vi "Write Parameters.vi"(8 "error in (no error)":errorcluster, 10 "Parameters":T1, 11 "PID in":refnum<class "PID.lvclass">) -> (0 "error out":errorcluster, 3 "PID out":refnum<class "PID.lvclass">)   [LabVIEW 2020, in "IG PID.lvlib" / "PID.lvclass"]
uses:
  PID.lvclass
  Parameters.ctl
  PID.lvclass/PID.ctl
  IG PID.lvlib
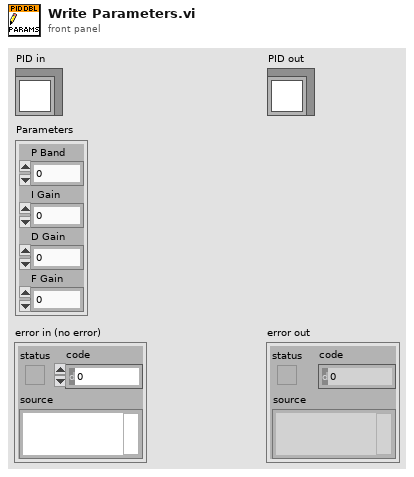
[diagram p1: front panel]
types:
  T1 = typedef "IG PID.lvlib/Parameters.ctl" = cluster{"P Band":dbl, "I Gain":dbl, "D Gain":dbl, "F Gain":dbl}
  T2 = typedef "IG PID.lvlib/Output Range.ctl" = cluster{"Min":dbl, "Max":dbl}
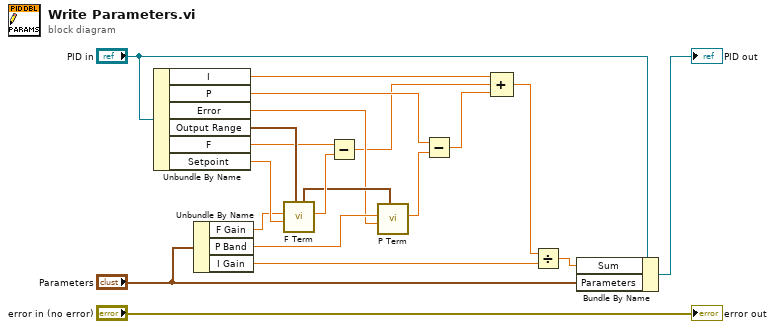
[diagram p0: block diagram]
diagram:
  n1 = Unbundle By Name("PID in") -> ("I"=w15:dbl, "P"=w3:dbl, "Error"=w5:dbl, "Output Range"=w10:T2, "F"=w9:dbl, "Setpoint"=w12:dbl)
  n2 = Unbundle By Name("Parameters") -> ("F Gain"=w11:dbl, "P Band"=w6:dbl, "I Gain"=w13:dbl)
  n3 = call "F Term.vi"("Output Range"=w10, "Setpoint"=w12, "F Gain"=w11) -> ("Output"=w8:dbl, "Remaining Range"=w7:T2)  [unwired: 7 in]
  n4 = Subtract(x=w9, y=w8) -> (x-y=w1:dbl)
  n5 = call "P Term.vi"("Output Range"=w7, "Error"=w5, "P Band"=w6) -> ("Output"=w4:dbl)  [unwired: 7 in, 1 out]
  n6 = Subtract(x=w3, y=w4) -> (x-y=w2:dbl)
  n7 = Compound Arithmetic op=ADD(w15, w1, w2) -> (w14:dbl)
  n8 = Divide(x=w14, y=w13) -> (x/y=w18:dbl)
  n9 = Bundle By Name(cluster="PID in", "Sum"=w18, "Parameters"="Parameters") -> (→"PID out":refnum<class "PID.lvclass">)
  "error out" <- "error in (no error)"
